vi "Init.vi"(8 "error in (no error)":errorcluster, 10 "Address":string, 11 "Inovance_Camera in":refnum<class "Inovance_Camera.lvclass">) -> (0 "error out":errorcluster, 3 "Inovance_Camera out":refnum<class "Inovance_Camera.lvclass">)   [LabVIEW 2023, in "Inovance_Camera.lvlib" / "Inovance_Camera.lvclass"]
uses:
  Inovance_Camera.lvclass
  C:/Program Files/National Instruments/LabVIEW 2023/vi.lib/ActorFramework/Actor/Actor.lvclass
  typedefs/AddressType.ctl
  typedefs/instrumentType.ctl
  <vilib>/userDefined/High Color/IMAQdx.ctl
  Inovance_Camera.lvclass/Inovance_Camera.ctl
  <vilib>/ActorFramework/Actor/Actor.lvclass/Actor.ctl
  Interfaces/InitDeinitInterface/InitDeinitComm Messages/InitDone Msg/InitDone Msg.lvclass/InitDone Msg.ctl
  <vilib>/ActorFramework/Message Enqueuer/Message Enqueuer.lvclass/Message Enqueuer.ctl
  Interfaces/AbstractInstrumentClasses/Cameras_LV/CameraComm Messages/Exposure Set Msg/Exposure Set Msg.lvclass/Exposure Set Msg.ctl
  <vilib>/ActorFramework/Message Enqueuer/Init from Existing Queue.vi
  <vilib>/ActorFramework/Message Enqueuer/Enqueue.vi
  Interfaces/InitDeinitInterface/InitDeinitComm Messages/InitDone Msg/InitDone Msg.lvclass
  C:/Program Files/National Instruments/LabVIEW 2023/vi.lib/ActorFramework/Message/Message.lvclass
  Interfaces/AbstractInstrumentClasses/Cameras_LV/CameraComm Messages/Exposure Set Msg/Exposure Set Msg.lvclass
  <vilib>/ActorFramework/Message Priority Queue/Priority Enqueue.vi
  <vilib>/ActorFramework/Message Enqueuer/Message Enqueuer.lvclass
  Inovance_Camera.lvlib
  typedefs/typedefs.lvlib
  <vilib>/ActorFramework/Actor/Actor.lvclass
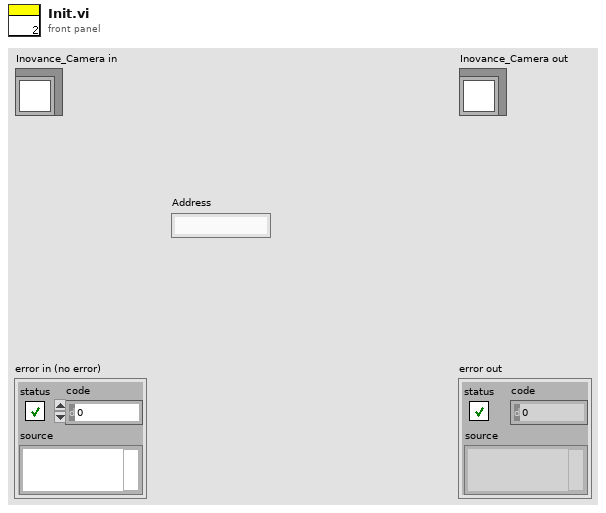
[diagram p1: front panel]
types:
  T1 = typedef "IMAQdx.ctl" = refnum<k21>
  T2 = typedef "typedefs.lvlib/instrumentType.ctl" = enum16{"Spectrometer", "Camera", "Stepper", "Piezo"}
  T3 = typedef "AddressType.ctl" = enum16{"VISA", "Index", "ModelNumber"}
  T4 = typedef "typedefs.lvlib/InstrumentData.ctl" = cluster{"Instr Error":errorcluster, "Address":cluster{"address type":enum16{"VISA", "Index"}, "Address":string, "instrument type":T2}, "CurrentState":cluster{"Initialized":bool, "Connected":bool, "Running":bool, "Error":bool}, "Enqueuer":refnum<class "Message Enqueuer.lvclass">}
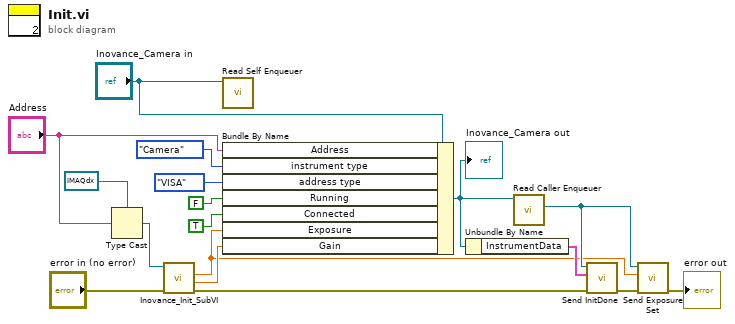
[diagram p0: block diagram]
diagram:
  n1 = Type Cast(type=T1 refnum ("Inovance Address"), x="Address") -> (*(type *) &x=w10:T1)
  n2 = call "Inovance_Init_SubVI.vi"("error in (no error)"="error in (no error)", "Inovance Address"=w10) -> ("error out"=w9:errorcluster, "Gain"=w5:dbl, "Exposure"=w1:dbl)  [unwired: 6 in, 1 out]
  n3 = call <vilib>:"Read Self Enqueuer.vi"("Actor"="Inovance_Camera in") -> ()  [unwired: 10 in, 1 out]
  n4 = Bundle By Name(cluster="Inovance_Camera in", "Address"="Address", "instrument type"=instrumentType."Camera" ("InstrumentData.Address.instrument type"), "address type"=AddressType."VISA" ("InstrumentData.Address.address type"), "Running"=FALSE ("InstrumentData.CurrentState.Running"), "Connected"=TRUE ("InstrumentData.CurrentState.Connected"), "Exposure"=w1, "Gain"=w5) -> (w13:refnum<class "Inovance_Camera.lvclass">)
  "Inovance_Camera out" <- w13
  n5 = Unbundle By Name(w13) -> ("InstrumentData"=w14:T4)
  n6 = call <vilib>:"Read Caller Enqueuer.vi"("Actor"=w13) -> ("Caller Enqueuer"=w4:refnum<class "Message Enqueuer.lvclass">)  [unwired: 10 in]
  n7 = call "Send InitDone.vi"("error in (no error)"=w9, "InstrumentData"=w14, "Message Enqueuer"=w4) -> ("error out"=w3:errorcluster)  [unwired: 7 in, 1 out]
  n8 = call "Send Exposure Set.vi"("error in (no error)"=w3, "Exposure(ms)"=w1, "Message Enqueuer"=w4) -> ("error out"=→"error out":errorcluster)  [unwired: 7 in, 1 out]
